vi "ParseGateInfo.vi"(9 "Gate Width":dbl, 10 "# Frames":i32, 11 "Gate Start":dbl) -> (2 "Numeric":dbl, 3 "Boolean":bool)   [LabVIEW 2018]
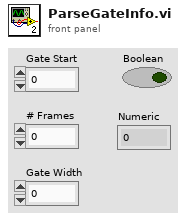
[diagram p1: front panel]
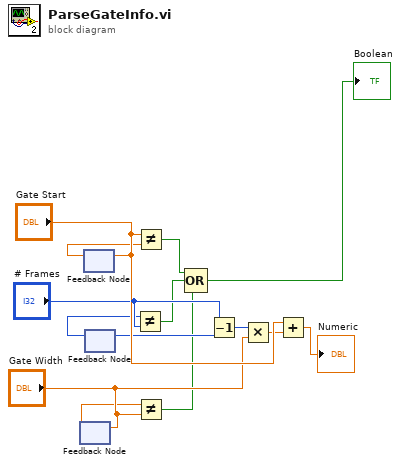
[diagram p0: block diagram]
diagram:
  n1 = feedback #1() -> (w7:dbl)  [unwired: 1 in]
  n2 = feedback-in #1("Gate Width") -> ()
  n3 = feedback #2() -> (w1:dbl)  [unwired: 1 in]
  n4 = feedback-in #2("Gate Start") -> ()
  n5 = feedback #3() -> (w6:i32)  [unwired: 1 in]
  n6 = feedback-in #3("# Frames") -> ()
  n7 = Not Equal?(x=w6, y="# Frames") -> (x != y?=w5:bool)
  n8 = Not Equal?(x="Gate Start", y=w1) -> (x != y?=w3:bool)
  n9 = Not Equal?(x=w7, y="Gate Width") -> (x != y?=w4:bool)
  n10 = Compound Arithmetic op=OR(w3, w5, w4) -> (→"Boolean":bool)
  n11 = Decrement(x="# Frames") -> (x-1=w9:i32)
  n12 = Multiply(x=w9, y="Gate Width") -> (x*y=w2:dbl)
  n13 = Add(x="Gate Start", y=w2) -> (x+y=→"Numeric":dbl)
